vi "create nthread engine.vi"(8 "error in":errorcluster, 11 "threadCount":u64=2) -> (0 "error out":errorcluster, 3 "engine":u64)   [LabVIEW 2016, in "async tls dl.lvlib"]
uses:
  async tls dl.lvlib
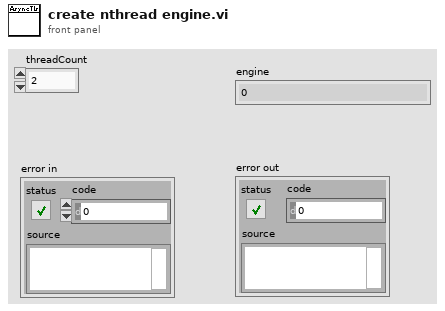
[diagram p1: front panel]
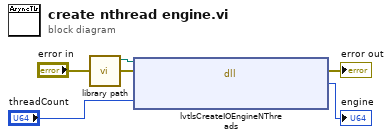
[diagram p0: block diagram]
diagram:
  n1 = call "library path.vi"() -> ("path"=w2:path)  [unwired: 11 in]
  n2 = dll-call lib="C:/Users/IEUser/Desktop/libasynclvtls/lvasynctls.dll" fn="lvtlsCreateIOEngineNThreads" ("lvasynctls.dll:lvtlsCreateIOEngine")(path in=w2, error in="error in", "threadCount"="threadCount") -> (error out=→"error out":errorcluster, "engine"=→"engine":u64)  [unwired: 2 in, 1 out]
